vi "Task Loop.vi"(8 "error in (no error)":errorcluster, 11 "ChartGuiTask in":refnum<class "ChartGuiTask.lvclass">) -> (0 "error out":errorcluster)   [LabVIEW 2020, in "VolatusDemo.lvlib" / "ChartGuiTask.lvclass"]
uses:
  ChartGuiTask.lvclass
  ChartGuiTask.lvclass/ChartGuiTask.ctl
panel:
  out "XY Graph":cluster{"X":dbl, "Y":dbl}[](graph)
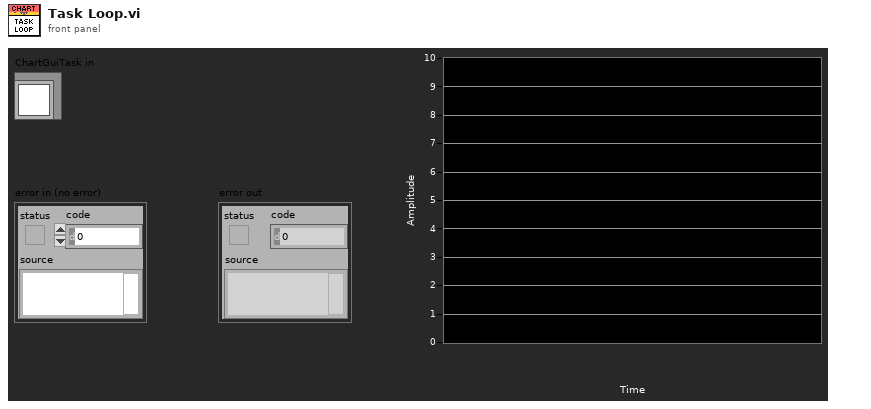
[diagram p1: front panel]
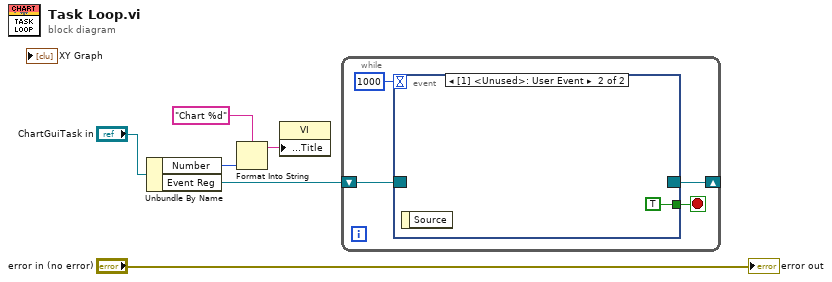
[diagram p0: block diagram]
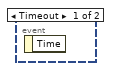
[diagram p2: hidden frame]
diagram:
  n1 = Unbundle By Name("ChartGuiTask in") -> ("Number"=w3:i32, "Event Reg"=w2:refnum<event-registration>)
  n2 = Format Into String(format string="Chart %d", w3) -> (resulting string=w1:string)  [unwired: 2 in, 1 out]
  n3 = property class="VI"("Front Panel.Title"=w1) -> ()  [unwired: 2 in, 2 out]
  n4 = while {
    shift-right: [w8] -> _
    shift-left: w2 -> [w9]
    stop <- w7 stop-if-true
    n5 = event shown="[1] <Unused>: User Event" {
      selector: w9 -> [_ _]
      dyn-events: [_ _] -> w8
      timeout: 1000 -> [_ _]
      tunnel: [_ TRUE] -> w7
      event Timeout {
        n6 = event-data() -> ()  [unwired: 1 in, 1 out]
      }
      event User Event {
        n7 = event-data() -> ()  [unwired: 1 in, 1 out]
      }
    }
  }
  "error out" <- "error in (no error)"
